vi "TabControl.vi"(0 "Page Visible":bool, 1 "whichPage":T1(ring), 2 "Tab Control":T2(tab)=enum."XY Intensity Map Acquisition") -> ()   [LabVIEW 2019]
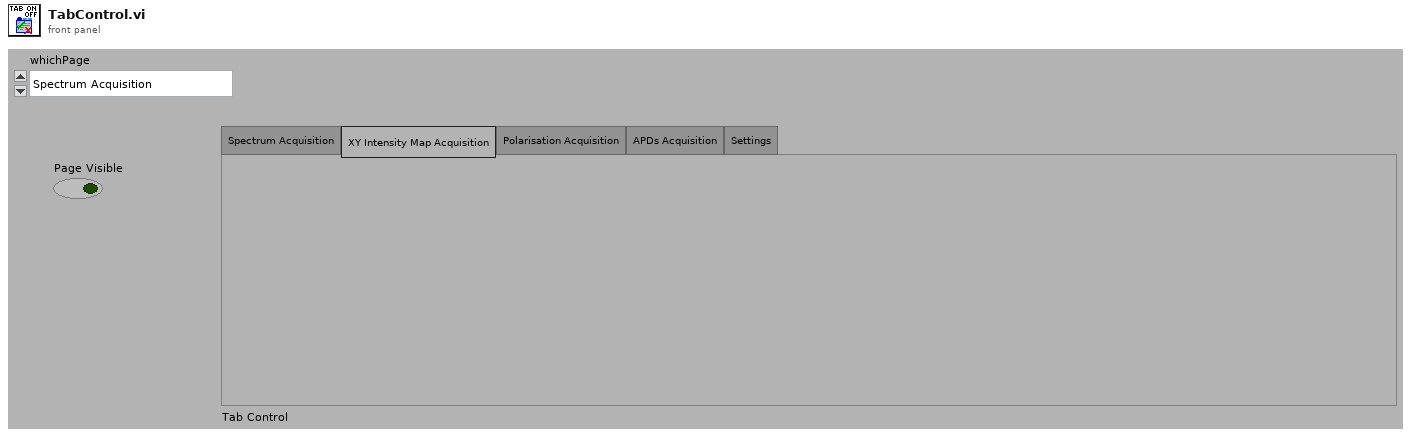
[diagram p1: front panel]
types:
  T1 = enum16{"Spectrum Acquisition", "XY Intensity Map Acquisition", "Polarisation Acquisition", "APDs Acquisition", "Settings"}
  T2 = enum32{"Spectrum Acquisition", "XY Intensity Map Acquisition", "Polarisation Acquisition", "APDs Acquisition", "Settings"}
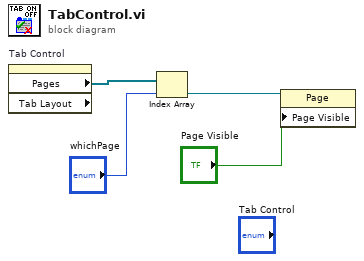
[diagram p0: block diagram]
diagram:
  n1 = property on="Tab Control" class="TabCtl (strict)" props=["Pages", "Tab Layout"]() -> ("Pages"=w4:refnum<vi>[])  [unwired: 2 in, 3 out]
  n2 = Index Array(array=w4, index="whichPage") -> (element=w3:refnum<vi>)
  n3 = property class="Page"(reference=w3, "Page Visible"="Page Visible") -> ()  [unwired: 1 in, 2 out]
